vi "Pre Launch Init.vi"(11 "Nested in":refnum<class "Monedas MXN.lvclass">) -> (0 "error out":errorcluster, 3 "Nested out":refnum<class "Monedas MXN.lvclass">)   [LabVIEW 2020, in "Monedas MXN.lvlib" / "Monedas MXN.lvclass"]
doc: "(<B>Filename</B>: Actor Framework.lvlib:Actor.lvclass:Pre Launch Init.vi)\n\nDefines behavior that occurs after the Launch Nested Actor method is invoked but before the actor's Actor Core method begins running.\n\nBy default, this method does nothing. A descendant class may override it to define behavior."
uses:
  Monedas MXN.lvclass
  C:/Program Files (x86)/National Instruments/LabVIEW 2020/vi.lib/ActorFramework/Actor/Actor.lvclass
  Monedas MXN.lvclass/Monedas MXN.ctl
  <vilib>/ActorFramework/Actor/Actor.lvclass/Actor.ctl
  <vilib>/ActorFramework/Message Enqueuer/Message Enqueuer.lvclass/Message Enqueuer.ctl
  <vilib>/ActorFramework/Message Enqueuer/Init from Existing Queue.vi
  <vilib>/ActorFramework/Message Enqueuer/Enqueue.vi
  Monedas MXN Messages/Init Msg/Init Msg.lvclass
  C:/Program Files (x86)/National Instruments/LabVIEW 2020/vi.lib/ActorFramework/Message/Message.lvclass
  <vilib>/ActorFramework/Message Priority Queue/Priority Enqueue.vi
  <vilib>/ActorFramework/Message Enqueuer/Message Enqueuer.lvclass
  <vilib>/ActorFramework/Actor/Actor.lvclass
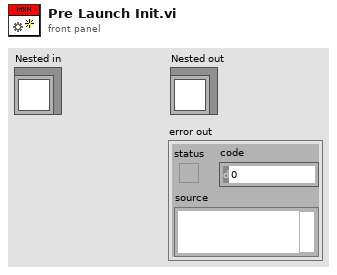
[diagram p1: front panel]
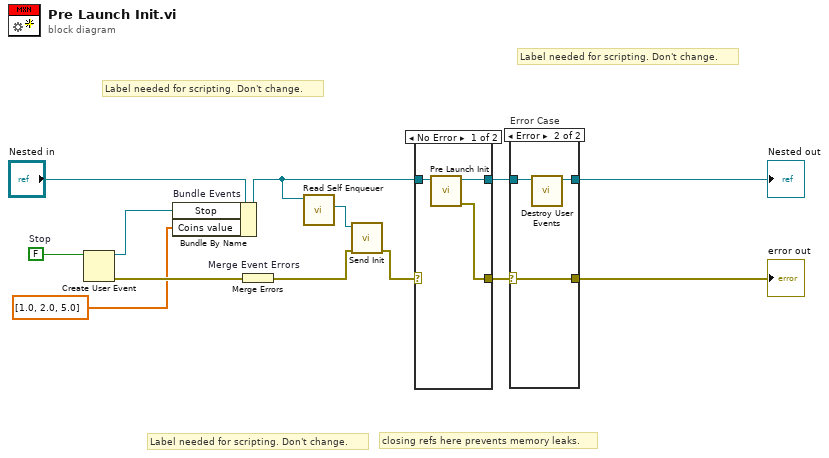
[diagram p0: block diagram]
diagram:
  w12 = FALSE  # Stop
  # "Label needed for scripting. Don't change."
  # "Label needed for scripting. Don't change."
  # "Label needed for scripting. Don't change."
  # "closing refs here prevents memory leaks."
  n1 = Create User Event(user event datatype=w12) -> (user event=w9:refnum<user-event>, error out=w11:errorcluster)  [unwired: 1 in]
  n2 = Bundle By Name "Bundle Events"(cluster="Nested in", "Stop"=w9, "Coins value"=dbl[] [1.0, 2.0, 5.0]) -> (w5:refnum<class "Monedas MXN.lvclass">)
  n3 = Merge Errors "Merge Event Errors"(w11) -> (w3:errorcluster)
  n4 = call <vilib>:"Read Self Enqueuer.vi"("Actor"=w5) -> ("Self Enqueuer"=w4:refnum<class "Message Enqueuer.lvclass">)  [unwired: 10 in]
  n5 = call "Send Init.vi"("error in (no error)"=w3, "Message Enqueuer"=w4) -> ("error out"=w2:errorcluster)  [unwired: 8 in, 1 out]
  n6 = case shown="No Error" w2 {
    selector: w2 -> [_ w18]
    tunnel: [w16 w17] -> w7
    tunnel: w5 -> [w15 w17]
    tunnel: [w14 w18] -> w6
    frame No Error {
      n7 = call-parent "Pre Launch Init.vi"("Actor in"=w15) -> ("error out"=w14:errorcluster, "Actor out"=w16:refnum<class "Monedas MXN.lvclass">)  [unwired: 9 in]
    }
    frame Error {
    }
  }
  n8 = case "Error Case" shown="Error" w6 {
    selector: w6 -> [w19 w23]
    tunnel: w7 -> [w20 w22]
    tunnel: [w20 w21] -> w10
    tunnel: [w19 w23] -> w8
    frame No Error {
    }
    frame Error {
      n9 = call "Destroy User Events.vi"("UI Template in"=w22) -> ("UI Template out"=w21:refnum<class "Monedas MXN.lvclass">)  [unwired: 10 in]
    }
  }
  "error out" <- w8
  "Nested out" <- w10
